vi "Error Reported.vi"(8 "error in (no error)":errorcluster, 9 "Additional Information":string, 10 "Error":errorcluster) -> (0 "error out":errorcluster)   [LabVIEW 2024, in "Anode.lvlib"]
doc: "Send the Error Reported event to any VI registered to listen to events from the owning module.\n_____\nBased on Delacor QMH Project Template 3.1.0.34.\n\n<b>Note:</b> This VI was modified by the <b>Validate DQMH Module</b> tool to parse additional information tags out of the incoming error source string.\n\n<b>Note:</b> This VI was modified by the <b>Validate DQMH Module</b> tool to have a broadcast event glyph overlay on its icon."
uses:
  Anode.lvlib
  Error Reported Argument--cluster.ctl
  <vilib>/Delacor/Delacor QMH/Libraries/Message Queue_class/Delacor_lib_QMH_Message Queue.lvclass
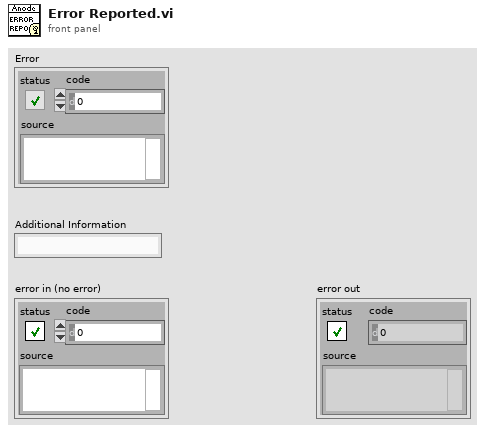
[diagram p1: front panel]
types:
  T1 = typedef "Anode.lvlib/Error Reported Argument--cluster.ctl" = cluster{"Error":errorcluster, "Additional Information":string, "Module Name":string}
  T2 = typedef "Anode.lvlib/Broadcast Events--cluster.ctl" = cluster{"Module Did Init":refnum<user-event>, "Status Updated":refnum<user-event>, "Error Reported":refnum<user-event>, "Module Did Stop":refnum<user-event>, "Update Module Execution Status":refnum<user-event>, "Broadcast Anode State":refnum<user-event>, "Broadcast H2 Sensor Data":refnum<user-event>}
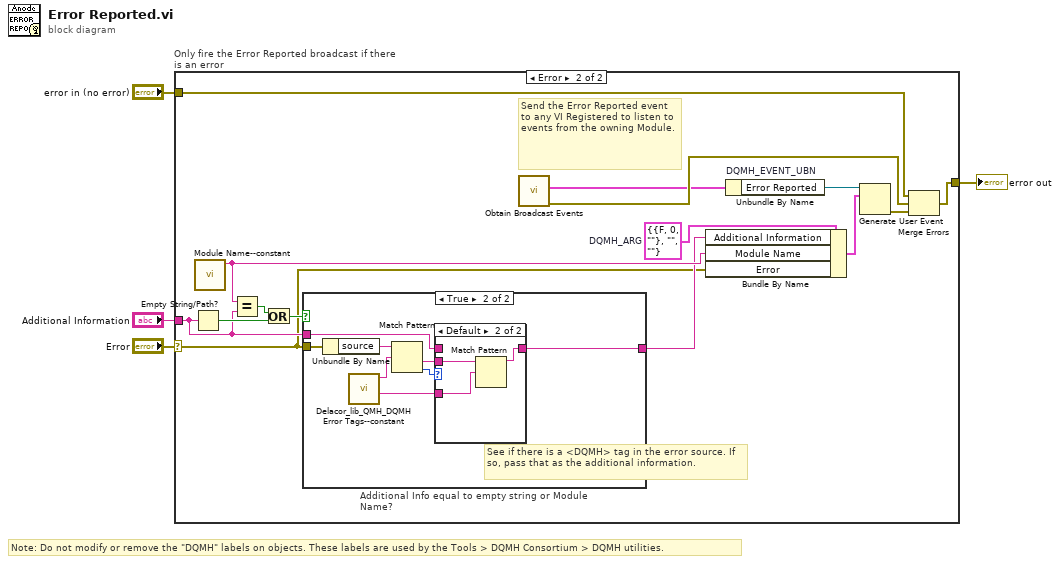
[diagram p0: block diagram]
diagram:
  # "Note: Do not modify or remove the \"DQMH\" labels on objects. These labels are used by the Tools > DQMH Consortium > DQMH utilities."
  n1 = case "Only fire the Error Reported broadcast if there is an error" shown="Error" "Error" {
    selector: "Error" -> [_ w8]
    tunnel: [w5 w20] -> w4
    tunnel: "error in (no error)" -> [w5 w6]
    tunnel: "Additional Information" -> [_ w10]
    frame No Error {
      # "No error was wired in, so don't fire the Error Reported broadcast."
    }
    frame Error {
      w16 = T1 {"Error"={"status"=FALSE, "code"=0, "source"=""}, "Additional Information"="", "Module Name"=""}  # DQMH_ARG
      # "Send the Error Reported event to any VI Registered to listen to events from the owning Module."
      n2 = Empty String/Path?(string/path=w10) -> (empty?=w12:bool)
      n3 = call "Module Name--constant.vi"() -> ("Module Name"=w14:string)  [unwired: 11 in]
      n4 = Equal?(x=w14, y=w10) -> (x = y?=w13:bool)
      n5 = Or(x=w13, y=w12) -> (x .or. y?=w11:bool)
      n6 = case "Additional Info equal to empty string or Module Name?" shown="True" w11 {
        tunnel: w10 -> [w21 w22]
        tunnel: [w21 w23] -> w9
        tunnel: w8 -> [_ w29]
        frame False {
          # "If the additional information string is not equal to empty string or module name, then the user has specified a custom string, and we should pass that value."
        }
        frame True {
          # "See if there is a <DQMH> tag in the error source. If so, pass that as the additional information."
          n7 = Unbundle By Name(w29) -> ("source"=w28:string)
          n8 = call <vilib>:"Delacor_lib_QMH_DQMH Error Tags--constant.vi"() -> ("Close Tag"=w24:string, "Open Tag"=w27:string)  [unwired: 10 in]
          n9 = Match Pattern(string=w28, regular expression=w27) -> (after substring=w25:string, offset past match=w26:i32)  [unwired: 1 in, 2 out]
          n10 = case shown="Default" w26 {
            tunnel: w25 -> [_ w33]
            tunnel: w24 -> [_ w32]
            tunnel: [w30 w31] -> w23
            tunnel: w22 -> [w30 _]
            frame -1 {
            }
            frame Default {
              n11 = Match Pattern(string=w33, regular expression=w32) -> (before substring=w31:string)  [unwired: 1 in, 3 out]
            }
          }
        }
      }
      n12 = call "Obtain Broadcast Events.vi"() -> ("error out"=w19:errorcluster, "Anode Broadcast Events"=w18:T2)  [unwired: 10 in]
      n13 = Bundle By Name(cluster=w16, "Additional Information"=w9, "Module Name"=w14, "Error"=w8) -> (w15:T1)
      n14 = Unbundle By Name "DQMH_EVENT_UBN"(w18) -> ("Error Reported"=w17:refnum<user-event>)
      n15 = Generate User Event(user event=w17, event data cluster=w15) -> (error out=w7:errorcluster)  [unwired: 2 in, 1 out]
      n16 = Merge Errors(w6, w19, w7) -> (w20:errorcluster)
    }
  }
  "error out" <- w4
